vi "spectra_voltage_read_txt.vi"(8 "VOLTAGE_PATH":path, 9 "Boolean ref in":refnum<vi>, 11 "SPECTRA_DIRECTORY":path) -> (0 "transmissions[r=wl, c=v]":dbl[][](array[numeric]), 2 "wavelengths":dbl[](array[numeric]), 3 "voltages":dbl[](array[numeric]), 5 "voltage file errors":errorcluster, 7 "spectra directory errors":errorcluster)   [LabVIEW 2019]
uses:
  <vilib>/Utility/file.llb/Read Delimited Spreadsheet (DBL).vi
  REFS.vi
panel:
  out "iteration":i32
  out "task size":i32
  # "Inputs (double click on folder icon)"
  # "Errors"
  # "Outputs"
  # "Error code d7 means that the selected file/folder does not exist.\nSee online labview documentation for other errors."
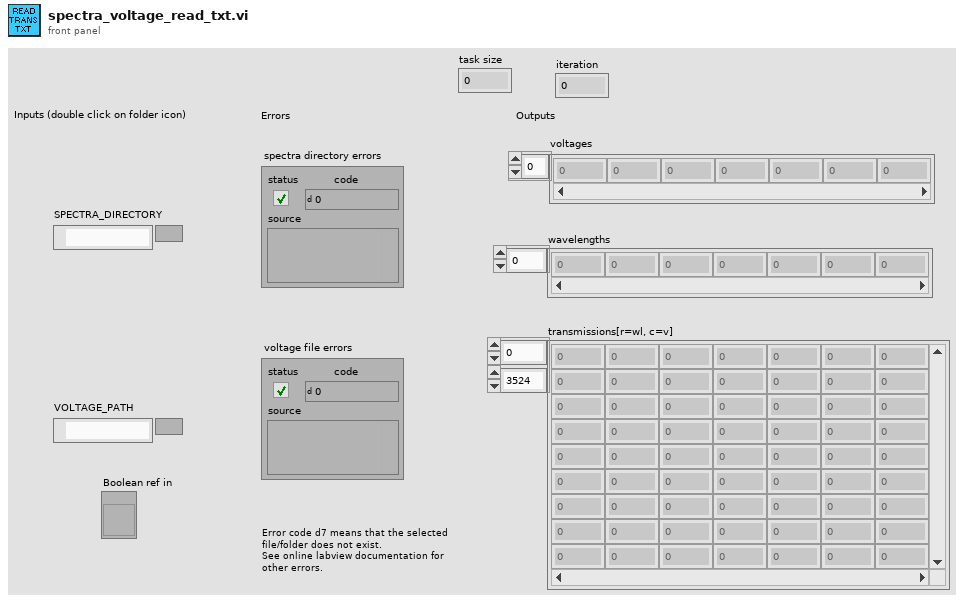
[diagram p1: front panel]
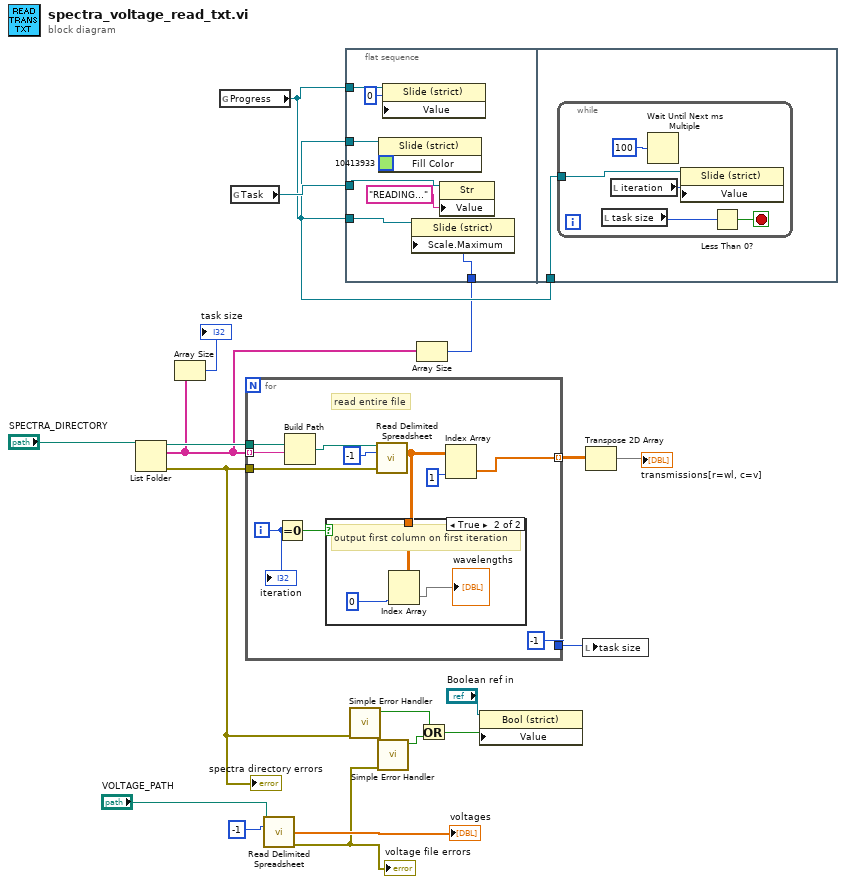
[diagram p0: block diagram]
diagram:
  n1 = List Folder(path="SPECTRA_DIRECTORY") -> (path out=w18:path, filenames=w12:string[], error out=w1:errorcluster)  [unwired: 3 in, 1 out]
  "spectra directory errors" <- w1
  n2 = Array Size(array=w12) -> (size(s)=→"task size":i32)
  n3 = global read "REFS.vi" "Progress"() -> (w3:refnum<vi>)
  n4 = global read "REFS.vi" "Task"() -> (w4:refnum<vi>)
  n5 = for {
    tunnel: w18 -> [w30]
    tunnel: w12 -> [w29] mode=indexing
    tunnel: w1 -> [w27]
    tunnel: [w20] -> w11 mode=indexing
    tunnel: [-1] -> w13
    i -> [w22]
    # "read entire file"
    n6 = Equal To 0?(x=w22) -> (x = 0?=w25:bool)
    n7 = Build Path(base path=w30, name or relative path=w29) -> (appended path=w28:path)
    n8 = call-poly <vilib>:"Read Delimited Spreadsheet.vi"("file path (dialog if empty)"=w28, "number of rows (all:-1)"=-1, "error in (no error)"=w27) -> ("all rows"=w24:dbl[][])  [unwired: 7 in, 5 out]
    n9 = case shown="True" w25 {
      tunnel: w24 -> [_ w33]
      frame False {
      }
      frame True {
        # "output first column on first iteration"
        n10 = Index Array "Index Array"(array=w33, index (col)=0) -> (element=→"wavelengths":dbl[])  [unwired: 1 in]
      }
    }
    n11 = Index Array "Index Array"(array=w24, index (col)=1) -> (element=w20:dbl[])  [unwired: 1 in]
    "iteration" <- w22
  }
  n12 = call-poly <vilib>:"Read Delimited Spreadsheet.vi"("file path (dialog if empty)"="VOLTAGE_PATH", "number of rows (all:-1)"=-1) -> ("first row"=→"voltages":dbl[], "error out"=w8:errorcluster)  [unwired: 8 in, 4 out]
  "voltage file errors" <- w8
  n13 = flat-sequence {
    tunnel: w3 -> [w38]
    tunnel: w3 -> [w37]
    tunnel: w4 -> [w36]
    tunnel: w3 -> [w35]
    tunnel: w2 -> [w34]
    tunnel: w3 -> [w42]
    frame #0 {
      n14 = property on="Property Node" class="Slide (strict)"(reference=w37, "Fill Color"=u32 10413933) -> ()  [unwired: 1 in, 2 out]
      n15 = property class="Slide (strict)"(reference=w38, "Value"=0) -> ()  [unwired: 1 in, 2 out]
      n16 = property on="Property Node" class="Slide (strict)"(reference=w35, "Scale.Maximum"=w34) -> ()  [unwired: 1 in, 2 out]
      n17 = property class="Str"(reference=w36, "Value"="READING...") -> ()  [unwired: 1 in, 2 out]
    }
    frame #1 {
      n18 = while {
        tunnel: w42 -> [w45]
        stop <- w46 stop-if-true
        n19 = local read "task size"() -> (w43:i32)
        n20 = local read "iteration"() -> (w44:i32)
        n21 = Wait Until Next ms Multiple(millisecond multiple=100) -> ()  [unwired: 1 out]
        n22 = property class="Slide (strict)"(reference=w45, "Value"=w44) -> ()  [unwired: 1 in, 2 out]
        n23 = Less Than 0?(x=w43) -> (x < 0?=w46:bool)
      }
    }
  }
  n24 = call <vilib>:"Simple Error Handler.vi"("error in (no error)"=w1) -> ("error?"=w7:bool)  [unwired: 4 in, 4 out]
  n25 = call <vilib>:"Simple Error Handler.vi"("error in (no error)"=w8) -> ("error?"=w6:bool)  [unwired: 4 in, 4 out]
  n26 = Array Size(array=w12) -> (size(s)=w2:i32)
  n27 = Or(x=w7, y=w6) -> (x .or. y?=w5:bool)
  n28 = property class="Bool (strict)"(reference="Boolean ref in", "Value"=w5) -> ()  [unwired: 1 in, 2 out]
  n29 = local write "task size"(w13) -> ()
  n30 = Transpose 2D Array(2D array=w11) -> (transposed array=→"transmissions[r=wl, c=v]":dbl[][])
